vi "HEWH Theoretical Draw Pattern.vi"(6 "Test Type":T1, 8 "error in (no error)":errorcluster, 11 "UEF Calculated Values Input":T2 {"Data Indexes"."15 sec after Draw Index" format="%#.2f"; "Data Indexes"."15 sec after Draw Timestamp" format="%#.2f"; "Data Indexes"."Test Start Timestamp" format="%.2f"; "Data Indexes"."Test End Timestamp" format="%.2f"; "Data Indexes"."T0 Timestamp" format="%.2f"; "Data Indexes"."Tsf Timestamp" format="%.2f"; "Data Indexes"."Tsu0 Timestamp" format="%.2f"; "Data Indexes"."Tmax1 Timestamp" format="%.2f"; "Data Indexes"."Draw Index Timestamp" format="%#.2f"; "Data Indexes"."Non-Draw Timestamp" format="%#.2f"; "Data Indexes"."Heating Timestamp" format="%#.2f"; "Data Indexes"."Start Energy (BTU-Gas)" format="%.6f"; "Data Indexes"."Start Watt Hours" format="%.6f"; "Static Data"."V - Volume of Wh (True)" format="%.5f"; "Static Data"."T-Ambinet Nominal (°F)" format="%.5f"; "Static Data"."T-Inlet Setpoint (°F)" format="%.5f"; "Static Data"."T-Wh Setpoint (°F)" format="%.5f"; "Sampled Data"."Qe (Wh)" format="%.5f"; "Sampled Data"."Tau stby2 (hr)" format="%.5f"; "Sampled Data"."Tastby2 (°F)" format="%.5f"; "Sampled Data"."Qf (BTU)" format="%.5f"; "Sampled Data"."Qe (BTU)" format="%.5f"; "Sampled Data"."Tmax1 (°F)" format="%.5f"; "Sampled Data"."T0 (°F)" format="%.5f"; "Sampled Data"."Qr (BTU)" format="%.5f"; "Sampled Data"."T 24(°F)" format="%.5f"; "Sampled Data"."T astby(°F)" format="%.5f"; "Sampled Data"."T tstby(°F)" format="%.5f"; "Sampled Data"."T su0(°F)" format="%.5f"; "Sampled Data"."T suf(°F)" format="%.5f"; "Sampled Data"."Tau stby_1 (hr)" format="%.5f"; "Sampled Data"."Qsuf (BTU)" format="%.5f"; "Sampled Data"."Qsu0 (BTU)" format="%.5f"; "Calculated Values"."Draw Bonus Volume (gal)" format="%.6f"; "Calculated Values"."Adjustment Factor" format="%.6f"; "Calculated Values"."T*avg_del(n-1)" format="%.6f"; "Calculated Values"."T*min(n-1)" format="%.6f"; "Calculated Values"."T*avg_del(n)" format="%.6f"; "Calculated Values"."Vn" format="%.6f"; "Calculated Values"."Qdm (BTU)" format="%.6f"; "Calculated Values"."QHWD (BTU)" format="%.6f"; "Calculated Values"."QHW (BTU)" format="%.6f"; "Calculated Values"."UEF" format="%.6f"; "Calculated Values"."QHW67 (BTU)" format="%.6f"; "Calculated Values"."Qda (BTU)" format="%.6f"; "Calculated Values"."Qd (BTU)" format="%.6f"; "Calculated Values"."Q (BTU)" format="%.6f"; "Calculated Values"."UA (BTU/(hr*F))" format="%.6f"; "Calculated Values"."Qhr (BTU/hr)" format="%.6f"; "Calculated Values"."Qstby (BTU)" format="%.6f"; "Calculated Values"."nu_r" format="%.6f"; "Calculated Values"."CpUEF (BTU/(lb*F))" format="%.6f"; "Calculated Values"."rho_nu (lb/gal)" format="%.6f"; "Calculated Values"."V1- Vol (Gal)" format="%.6f"; "Calculated Values"."M cluster mass removed (lb)" format="%.6f"; "Calculated Values"."Cp theoretical (BTU/(lbm °F))" format="%.6f"; "Calculated Values"."Tin1 - Mean Inlet 1st Cluster (°F)" format="%.6f"; "Calculated Values"."Tdel1-Mean Outlet 1st Cluster(°F)" format="%.6f"; "Calculated Values"."Cp 24 (BTU/(lb*F))" format="%.6f"; "Calculated Values"."Cp standby (BTU/(lb*F))" format="%.6f"; "Calculated Values"."Cp2 (BTU/(lb*F))" format="%.6f"; "Calculated Values"."Cp1 (BTU/(lb*F))" format="%.6f"; "Calculated Values"."rho 24 (lb/gal)" format="%.6f"; "Calculated Values"."rho standby (lb/gal)" format="%.6f"; "Calculated Values"."rho 2 (lb/gal)" format="%.6f"; "Calculated Values"."Density of cold water All (lbm/gal)" format="%#.3g"; "Calculated Values"."CpHW (BTU/(lbm °F))" format="%#.3g"; "Calculated Values"."Density of hot water All (lbm/gal)" format="%#.3g"; "Calculated Values"."Mass of water All (lbm)" format="%#.3f"}) -> (0 "error out":errorcluster, 3 "Theoretical Draw Pattern":dbl[][](array[numeric]))   [LabVIEW 2023]
uses:
  Type Definitions/UEF Constants.ctl
  Type Definitions/HEWH Draw Stats.ctl
  Type Definitions/HEWH FHR Draw Type.ctl
  Type Definitions/FHR Bins.ctl
  Type Definitions/HEWH Meter Type.ctl
  Type Definitions/HEWH Test Type.ctl
panel:
  # "FHR"
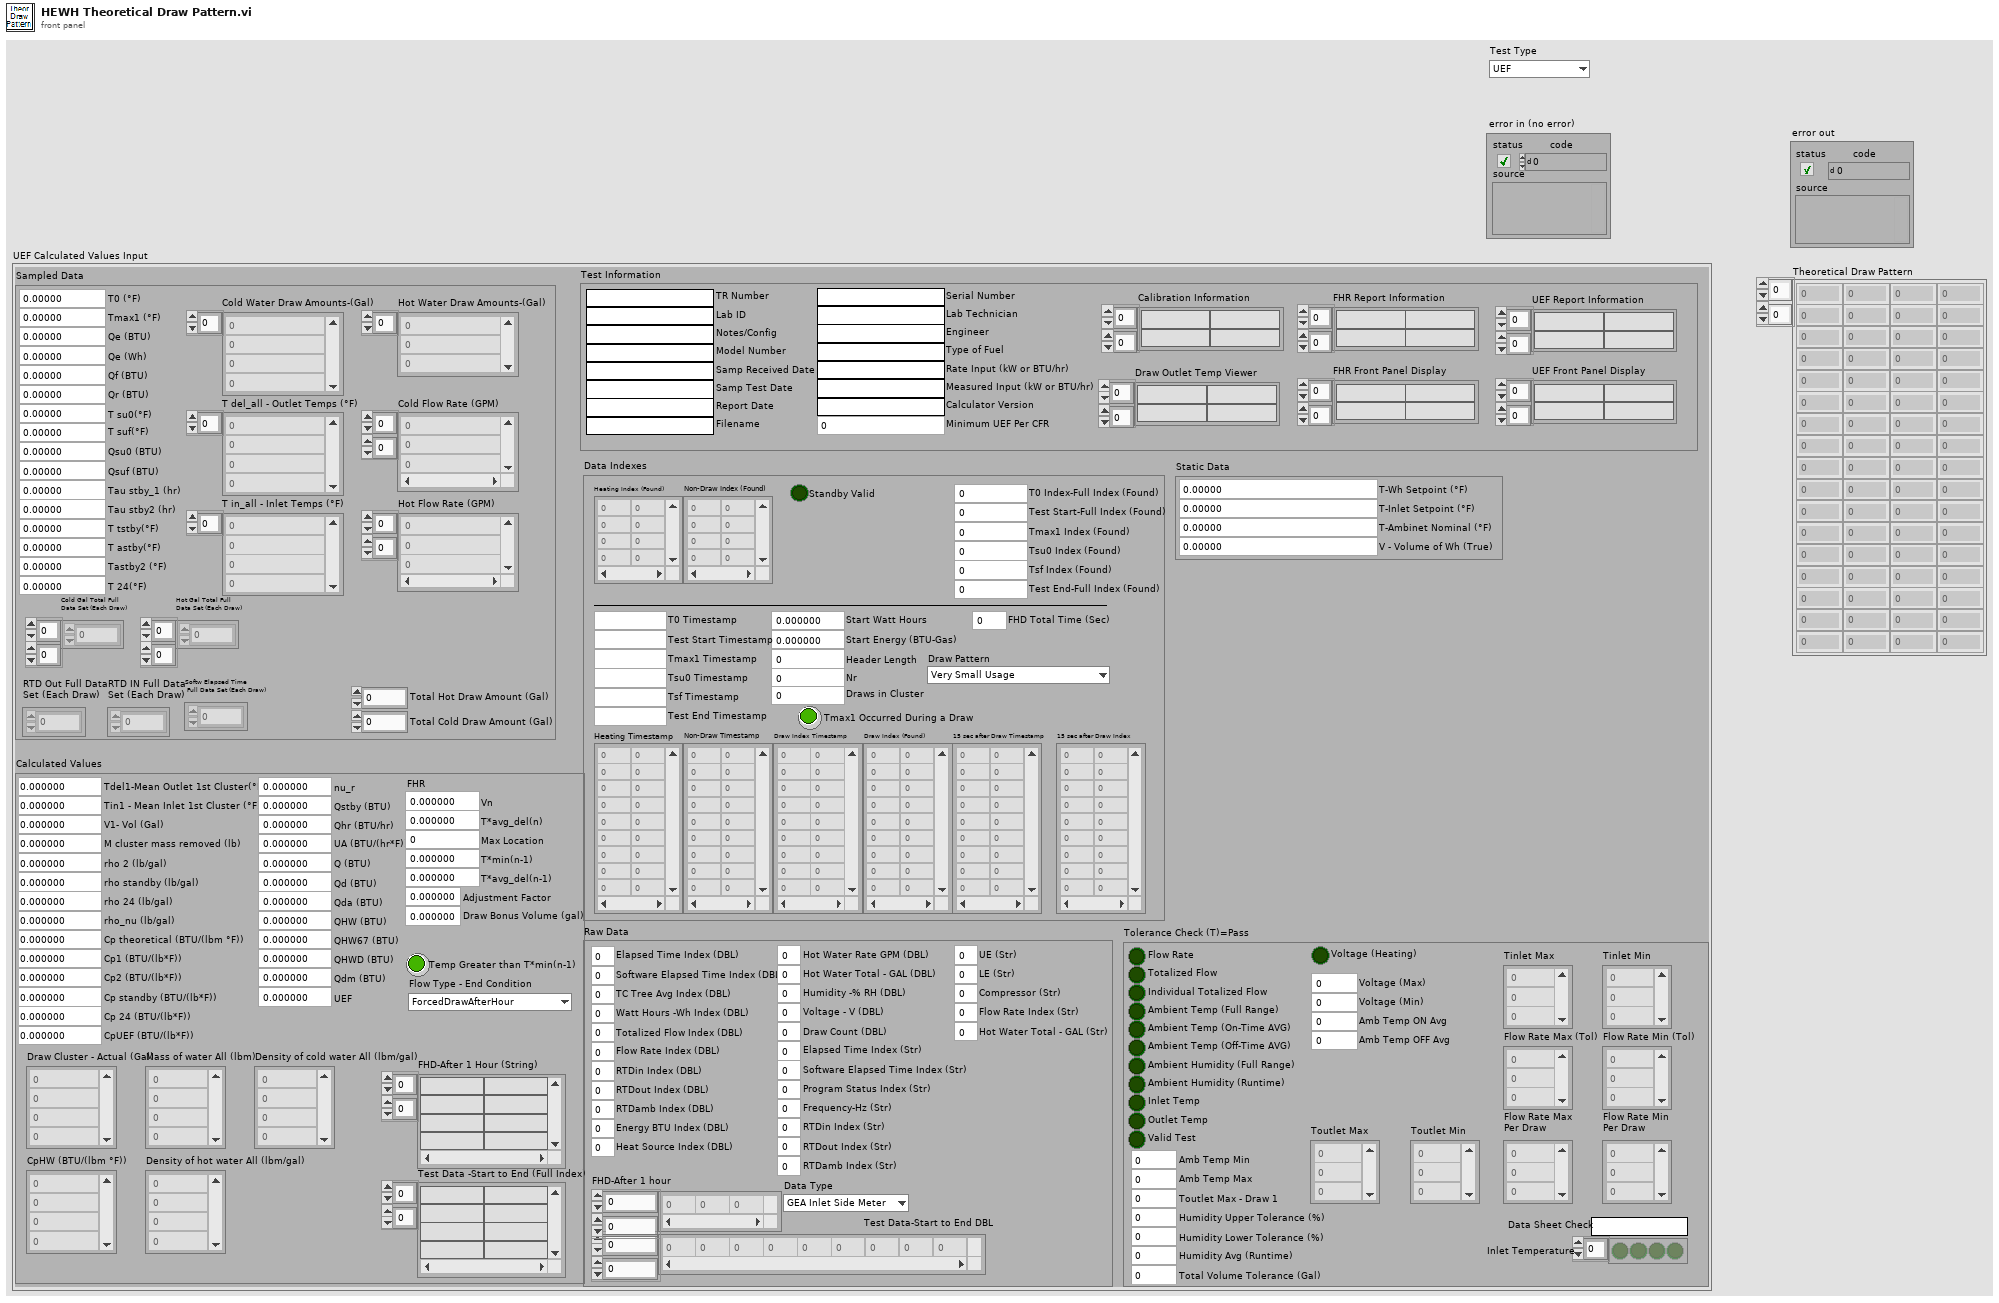
[diagram p1: front panel]
types:
  T1 = typedef "HEWH Test Type.ctl" = enum16{"UEF", "FHD"}
  T2 = typedef "UEF Constants.ctl" = cluster{"Calculated Values":T3, "Sampled Data":cluster{"Cold Water Draw Amounts-(Gal)":dbl[], "T del_all - Outlet Temps (°F)":dbl[], "T in_all - Inlet Temps (°F)":dbl[], "Qsu0 (BTU)":dbl, "Qsuf (BTU)":dbl, "Tau stby_1 (hr)":dbl, "T suf(°F)":dbl, "T su0(°F)":dbl, "T tstby(°F)":dbl, "T astby(°F)":dbl, "T 24(°F)":dbl, "Qr (BTU)":dbl, "T0 (°F)":dbl, "Tmax1 (°F)":dbl, "Qe (BTU)":dbl, "Qf (BTU)":dbl, "Tastby2 (°F)":dbl, "RTD Out Full Data\nSet (Each Draw)":dbl[][], "RTD IN Full Data\nSet (Each Draw)":dbl[][], "Tau stby2 (hr)":dbl, "Hot Water Draw Amounts-(Gal)":dbl[], "Cold Flow Rate (GPM)":dbl[][], "Hot Flow Rate (GPM)":dbl[][], "Softw Elapsed Time\n Full Data Set (Each Draw)":dbl[][], "Cold Gal Total Full\nData Set (Each Draw)":dbl[][], "Total Hot Draw Amount (Gal) ":dbl, "Total Cold Draw Amount (Gal)":dbl, "Qe (Wh)":dbl, "Hot Gal Total Full\nData Set (Each Draw)":dbl[][]}, "Static Data":cluster{"T-Wh Setpoint (°F)":dbl, "T-Inlet Setpoint (°F)":dbl, "T-Ambinet Nominal (°F)":dbl, "V - Volume of Wh (True)":dbl}, "Data Indexes":cluster{"Test Start-Full Index (Found)":i32, "Header Length":i32, "Draw Index (Found)":i32[][], "Nr":i32, "Start Watt Hours":dbl, "Tsu0 Index (Found)":i32, "Tsf Index (Found)":i32, "Start Energy (BTU-Gas)":dbl, "Draws in Cluster":i32, "T0 Index-Full Index (Found)":i32, "Non-Draw Index (Found)":i32[][], "Tmax1 Index (Found)":i32, "Test End-Full Index (Found)":i32, "Heating Index (Found)":i32[][], "Heating Timestamp":dbl[][], "Non-Draw Timestamp":dbl[][], "Draw Index Timestamp":dbl[][], "Tmax1 Timestamp":dbl, "Tsu0 Timestamp":dbl, "Tsf Timestamp":dbl, "T0 Timestamp":dbl, "Test End Timestamp":dbl, "Test Start Timestamp":dbl, "15 sec after Draw Timestamp":dbl[][], "15 sec after Draw Index":dbl[][], "Tmax1 Occurred During a Draw":bool, "FHD Total Time (Sec)":dbl, "Draw Pattern":T5, "Standby Valid":bool}, "Raw Data":cluster{"Elapsed Time Index (DBL)":i32, "Software Elapsed Time Index (DBL)":i32, "TC Tree Avg Index (DBL)":i32, "Watt Hours -Wh Index (DBL)":i32, "Energy BTU Index (DBL)":i32, "Totalized Flow Index (DBL)":i32, "Flow Rate Index (DBL)":i32, "Program Status Index (Str)":i32, "RTDin Index (DBL)":i32, "RTDout Index (DBL)":i32, "RTDamb Index (DBL)":i32, "Test Data-Start to End DBL":dbl[][], "Data Type":T6, "Heat Source Index (DBL)":i32, "Hot Water Rate GPM (DBL)":i32, "Hot Water Total - GAL (DBL)":i32, "FHD-After 1 hour":dbl[][], "Humidity -% RH (DBL)":i32, "Voltage - V (DBL)":i32, "Draw Count (DBL)":i32, "Elapsed Time Index (Str)":i32, "Software Elapsed Time Index (Str)":i32, "Frequency-Hz (Str)":i32, "RTDin Index (Str)":i32, "RTDout Index (Str)":i32, "RTDamb Index (Str)":i32, "UE (Str)":i32, "LE (Str)":i32, "Compressor (Str)":i32, "Flow Rate Index (Str)":i32, "Hot Water Total - GAL (Str)":i32}, "Tolerance Check (T)=Pass":cluster{"Flow Rate":bool, "Totalized Flow":bool, "Ambient Temp (Full Range)":bool, "Ambient Humidity (Full Range)":bool, "Inlet Temp":bool, "Outlet Temp":bool, "Valid Test":bool, "Individual Totalized Flow":bool, "Data Sheet Check":string, "Inlet Temperature":bool[], "Tinlet Max":dbl[], "Tinlet Min":dbl[], "Flow Rate Max (Tol)":dbl[], "Flow Rate Min (Tol)":dbl[], "Amb Temp Max":dbl, "Amb Temp Min":dbl, "Toutlet Max - Draw 1":dbl, "Humidity Upper Tolerance (%)":dbl, "Total Volume Tolerance (Gal)":dbl, "Humidity Lower Tolerance (%)":dbl, "Flow Rate Max\nPer Draw":dbl[], "Flow Rate Min\nPer Draw":dbl[], "Ambient Humidity (Runtime)":bool, "Humidity Avg (Runtime)":dbl, "Ambient Temp (On-Time AVG)":bool, "Ambient Temp (Off-Time AVG)":bool, "Amb Temp OFF Avg":dbl, "Amb Temp ON Avg":dbl, "Voltage (Heating)":bool, "Voltage (Min)":dbl, "Voltage (Max)":dbl, "Toutlet Max":dbl[], "Toutlet Min":dbl[]}, "Test Information":cluster{"TR Number":string, "Lab ID":string, "Notes/Config":string, "Model Number":string, "Serial Number":string, "Lab Technician":string, "Engineer":string, "Type of Fuel":string, "Samp Received Date":string, "Samp Test Date":string, "Report Date":string, "Rate Input (kW or BTU/hr)":string, "Measured Input (kW or BTU/hr)":string, "Filename":string, "Calibration Information":string[][], "Calculator Version":string, "Minimum UEF Per CFR":dbl, "UEF Report Information":string[][], "FHR Report Information":string[][], "FHR Front Panel Display":string[][], "UEF Front Panel Display":string[][], "Draw Outlet Temp Viewer":string[][]}}
  T3 = typedef "HEWH Draw Stats.ctl" = cluster{"Draw Cluster - Actual (Gal)":dbl[], "Mass of water All (lbm)":dbl[], "Density of hot water All (lbm/gal)":dbl[], "CpHW (BTU/(lbm °F))":dbl[], "rho 2 (lb/gal)":dbl, "rho standby (lb/gal)":dbl, "rho 24 (lb/gal)":dbl, "Cp1 (BTU/(lb*F))":dbl, "Cp2 (BTU/(lb*F))":dbl, "Cp standby (BTU/(lb*F))":dbl, "Cp 24 (BTU/(lb*F))":dbl, "nu_r":dbl, "Qstby (BTU)":dbl, "Qhr (BTU/hr)":dbl, "UA (BTU/(hr*F))":dbl, "Q (BTU)":dbl, "Qd (BTU)":dbl, "Qda (BTU)":dbl, "QHW67 (BTU)":dbl, "UEF":dbl, "Tdel1-Mean Outlet 1st Cluster(°F)":dbl, "Tin1 - Mean Inlet 1st Cluster (°F)":dbl, "Cp theoretical (BTU/(lbm °F))":dbl, "M cluster mass removed (lb)":dbl, "V1- Vol (Gal)":dbl, "Test Data -Start to End (Full Index)":string[][], "rho_nu (lb/gal)":dbl, "Density of cold water All (lbm/gal)":dbl[], "CpUEF (BTU/(lb*F))":dbl, "QHW (BTU)":dbl, "QHWD (BTU)":dbl, "Qdm (BTU)":dbl, "FHD-After 1 Hour (String)":string[][], "Vn":dbl, "T*avg_del(n)":dbl, "Max Location":i32, "T*min(n-1)":dbl, "T*avg_del(n-1)":dbl, "Temp Greater than T*min(n-1)":bool, "Adjustment Factor":dbl, "Draw Bonus Volume (gal)":dbl, "Flow Type - End Condition":T4}
  T4 = typedef "HEWH FHR Draw Type.ctl" = enum16{"ForcedDrawAfterHour", "HeatingCutoffBeforeHour"}
  T5 = typedef "FHR Bins.ctl" = enum16{"Very Small Usage", "Low Usage", "Medium Usage", "High Usage", "Undefined"}
  T6 = typedef "HEWH Meter Type.ctl" = enum16{"GEA Inlet Side Meter", "GEA Outlet Side Meter", "CSA Inlet Side Meter"}
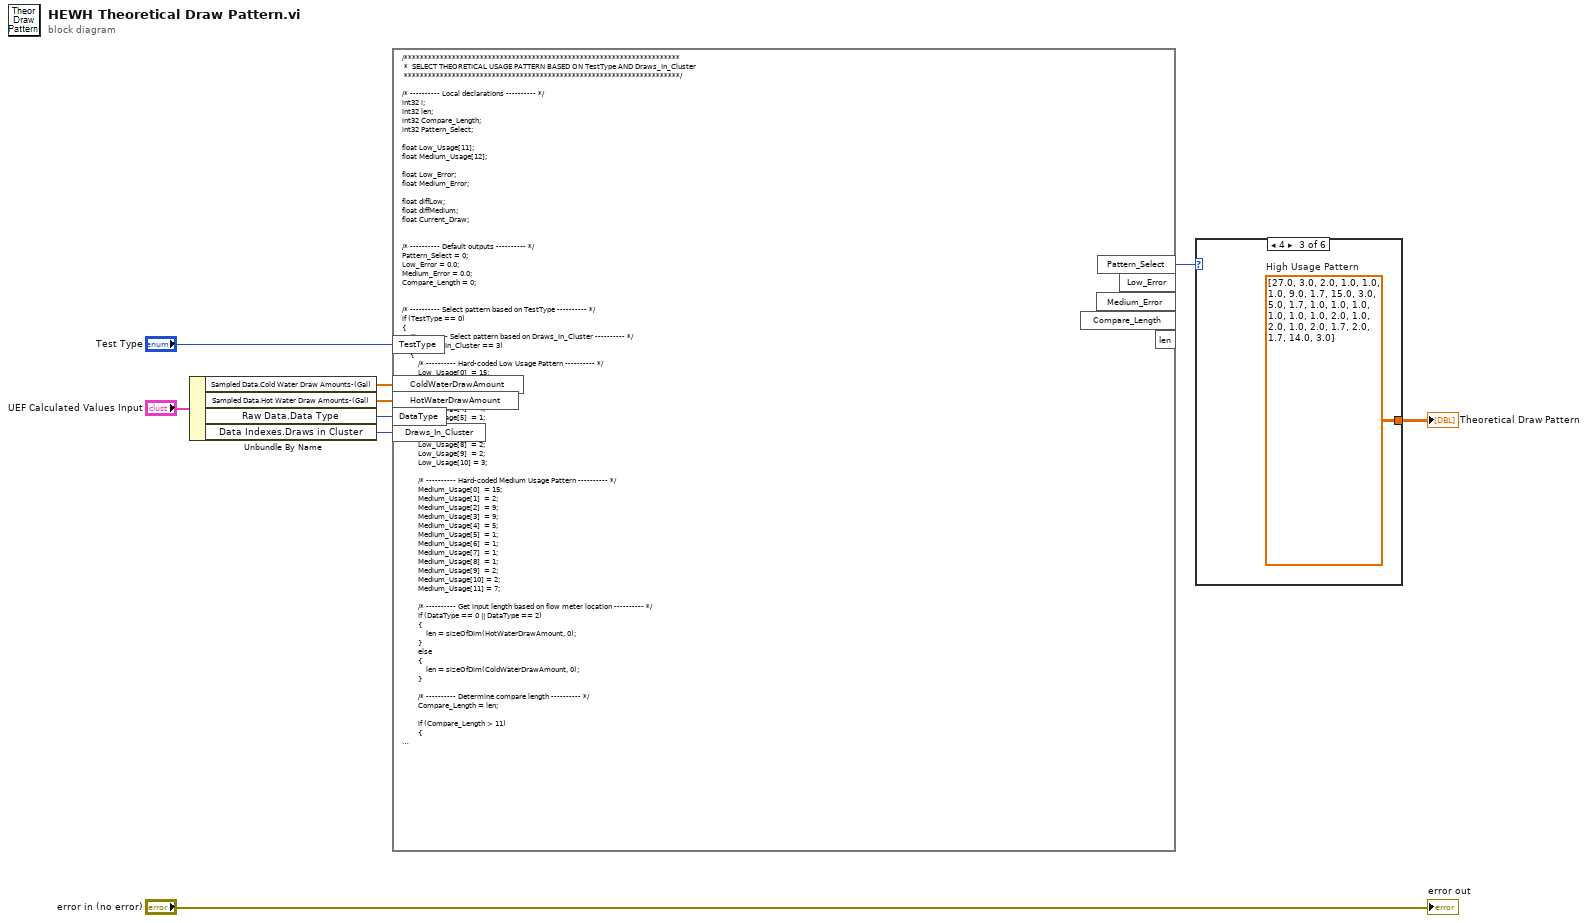
[diagram p0: block diagram]
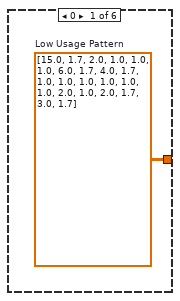
[diagram p2: hidden frame]
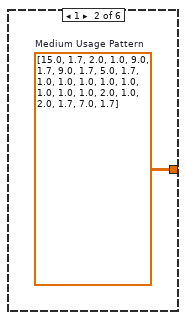
[diagram p3: hidden frame]
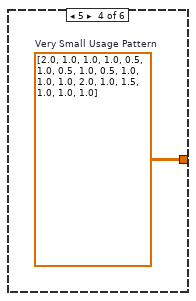
[diagram p4: hidden frame]
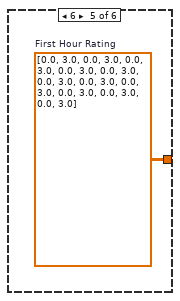
[diagram p5: hidden frame]
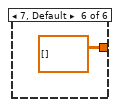
[diagram p6: hidden frame]
diagram:
  n1 = Unbundle By Name("UEF Calculated Values Input") -> ("Sampled Data.Cold Water Draw Amounts-(Gal)"=w4:dbl[], "Sampled Data.Hot Water Draw Amounts-(Gal)"=w3:dbl[], "Raw Data.Data Type"=w2:T6, "Data Indexes.Draws in Cluster"=w1:i32)
  n2 = formula code="/*********************************************************************\n *  SELECT THEORETICAL USAGE PATTERN BASED ON TestType AND Draws_In_Cluster\n *********************************************************************/\n\n/* ---------- Local declarations ---------- */\nint32 i;\nint32 len;\nint32 Compare_Length;\nint32 Pattern_Select;\n\nfloat Low_Usage[11];\nfloat Medium_Usage[12];\n\nfloat Low_Error;\nfloat Medium_Error;\n\nfloat diffLow;\nfloat diffMedium;\nfloat Current_Draw;\n\n\n/* ---------- Default outputs ---------- */\nPattern_Select = 0;\nLow_Error = 0.0;\nMedium_Error = 0.0;\nCompare_Length = 0;\n\n\n/* ---------- Select pattern based on TestType ---------- */\nif (TestType == 0)\n{\n    /* ---------- Select pattern based on Draws_In_Cluster ---------- */\n    if (Draws_In_Cluster == 3)\n    {\n        /* ---------- Hard-coded Low Usage Pattern ---------- */\n        Low_Usage[0]  = 15;\n        Low_Usage[1]  = 2;\n        Low_Usage[2]  = 1;\n        Low_Usage[3]  = 6;\n        Low_Usage[4]  = 4;\n        Low_Usage[5]  = 1;\n        Low_Usage[6]  = 1;\n        Low_Usage[7]  = 1;\n        Low_Usage[8]  = 2;\n        Low_Usage[9]  = 2;\n        Low_Usage[10] = 3;\n\n        /* ---------- Hard-coded Medium Usage Pattern ---------- */\n        Medium_Usage[0]  = 15;\n        Medium_Usage[1]  = 2;\n        Medium_Usage[2]  = 9;\n        Medium_Usage[3]  = 9;\n        Medium_Usage[4]  = 5;\n        Medium_Usage[5]  = 1;\n        Medium_Usage[6]  = 1;\n        Medium_Usage[7]  = 1;\n        Medium_Usage[8]  = 1;\n        Medium_Usage[9]  = 2;\n        Medium_Usage[10] = 2;\n        Medium_Usage[11] = 7;\n\n        /* ---------- Get input length based on flow meter location ---------- */\n        if (DataType == 0 || DataType == 2)\n        {\n            len = sizeOfDim(HotWaterDrawAmount, 0);\n        }\n        else\n        {\n            len = sizeOfDim(ColdWaterDrawAmount, 0);\n        }\n\n        /* ---------- Determine compare length ---------- */\n        Compare_Length = len;\n\n        if (Compare_Length > 11)\n        {\n            Compare_Length = 11;\n        }\n\n        /* ---------- Compute total absolute error ---------- */\n        for (i = 0; i < Compare_Length; i++)\n        {\n            if (DataType == 0 || DataType == 2)\n            {\n                Current_Draw = HotWaterDrawAmount[i];\n            }\n            else\n            {\n                Current_Draw = ColdWaterDrawAmount[i];\n            }\n\n            diffLow    = abs(Current_Draw - Low_Usage[i]);\n            diffMedium = abs(Current_Draw - Medium_Usage[i]);\n\n            Low_Error    = Low_Error + diffLow;\n            Medium_Error = Medium_Error + diffMedium;\n        }\n\n        /* ---------- Choose the closer pattern ---------- */\n        if (Medium_Error < Low_Error)\n        {\n            Pattern_Select = 1;    /* Medium Usage */\n        }\n        else\n        {\n            Pattern_Select = 0;    /* Low Usage */\n        }\n    }\n    else if (Draws_In_Cluster == 4)\n    {\n        Pattern_Select = 4;        /* High Usage */\n    }\n    else if (Draws_In_Cluster == 5)\n    {\n        Pattern_Select = 5;        /* Very Small Usage */\n    }\n    else\n    {\n        Pattern_Select = 7;        /* Default */\n    }\n}\nelse if (TestType == 1)\n{\n    Pattern_Select = 6;            /* First Hour Delivery */\n}\nelse\n{\n    Pattern_Select = 7;            /* Default */\n}"("Draws_In_Cluster"=w1, "TestType"="Test Type", "ColdWaterDrawAmount"=w4, "HotWaterDrawAmount"=w3, "DataType"=w2) -> ("Pattern_Select"=w6:i32)  [unwired: 4 out]
  n3 = case shown="4" w6 {
    tunnel: [w10 w11 w12 w13 w14 dbl[][] [] ("Very Small Usage Pattern")] -> w9
    frame 0 {
      w10 = dbl[][] [[15.0, 1.7], [2.0, 1.0], [1.0, 1.0], [6.0, 1.7], [4.0, 1.7], [1.0, 1.0], [1.0, 1.0], [1.0, 1.0], [2.0, 1.0], [2.0, 1.7], [3.0, 1.7]]  # Low Usage Pattern
    }
    frame 1 {
      w11 = dbl[][] [[15.0, 1.7], [2.0, 1.0], [9.0, 1.7], [9.0, 1.7], [5.0, 1.7], [1.0, 1.0], [1.0, 1.0], [1.0, 1.0], [1.0, 1.0], [2.0, 1.0], [2.0, 1.7], [7.0, 1.7]]  # Medium Usage Pattern
    }
    frame 4 {
      w12 = dbl[][] [[27.0, 3.0], [2.0, 1.0], [1.0, 1.0], [9.0, 1.7], [15.0, 3.0], [5.0, 1.7], [1.0, 1.0], [1.0, 1.0], [1.0, 1.0], [2.0, 1.0], [2.0, 1.0], [2.0, 1.7], [2.0, 1.7], [14.0, 3.0]]  # High Usage Pattern
    }
    frame 5 {
      w13 = dbl[][] [[2.0, 1.0], [1.0, 1.0], [0.5, 1.0], [0.5, 1.0], [0.5, 1.0], [1.0, 1.0], [2.0, 1.0], [1.5, 1.0], [1.0, 1.0]]  # Very Small Usage Pattern
    }
    frame 6 {
      w14 = dbl[][] [[0.0, 3.0], [0.0, 3.0], [0.0, 3.0], [0.0, 3.0], [0.0, 3.0], [0.0, 3.0], [0.0, 3.0], [0.0, 3.0], [0.0, 3.0], [0.0, 3.0], [0.0, 3.0]]  # First Hour Rating
    }
    frame 7, Default {
    }
  }
  "Theoretical Draw Pattern" <- w9
  "error out" <- "error in (no error)"
